vi "ustalRuchPionowy.vi"(6 "Kąt uśredniony":i32, 9 "Wybór komory":T3, 10 "Lista punktów w pionie":i32[](array[numeric]), 11 "Faza ruchu wstepna":T2) -> (2 "Stan pionowy":T1, 3 "Faza ruchu poziomego":T2)   [LabVIEW 2014]
uses:
  parametryKomorVIs/WyborKomory.ctl
  Faza_ruchu.ctl
  RuchPionowy.ctl
  AkcjaGFV.ctl
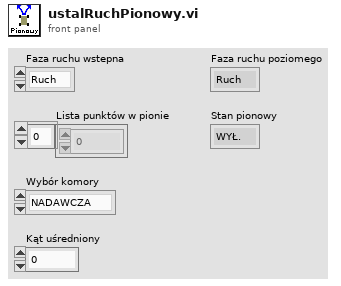
[diagram p1: front panel]
types:
  T1 = typedef "RuchPionowy.ctl" = enum16{"WYŁ.", "GÓRA", "Dӣ", "PRACA RĘCZNA"}
  T2 = typedef "Faza_ruchu.ctl" = enum16{"Ruch", "Poczekaj", "Pomiar"}
  T3 = typedef "WyborKomory.ctl" = enum16{"NADAWCZA", "ODBIORCZA"}
  T4 = typedef "WejsciaParametry.ctl" = cluster{"LEWO":bool, "PRAWO":bool, "GORA":bool, "DOL":bool, "Praca reczna":bool, "Stop":bool, "Start":bool, "Komora":bool, "Wyjscie":bool, "Rodzaj pomiarow":T5, "Czas pomiaru [s]":dbl, "Czas inicjalizacji ramion [s]":dbl, "Liczba punktów":i32, "Liczba płaszczyzn":i32}
  T5 = typedef "RodzajPomiarow.ctl" = enum16{"Izolacyjność Akustyczna ISO 10140", "Losowanie punktów", "Sekwencja testowa"}
  T6 = typedef "AkcjaGFV.ctl" = enum16{"Czytaj", "Zapisz", "Reset"}
  T7 = typedef "Gotowosc.ctl" = cluster{"Poziomy":bool, "Pionowy":bool}
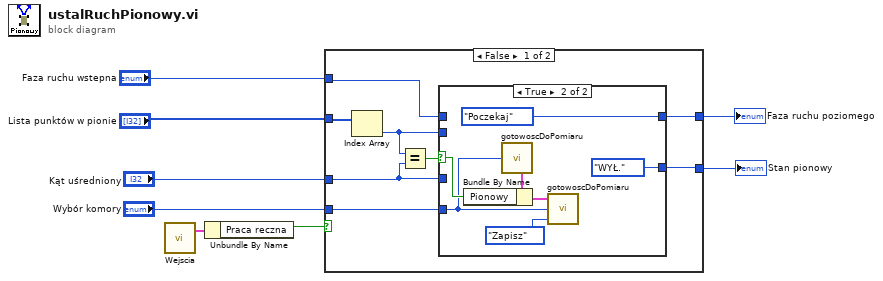
[diagram p0: block diagram]
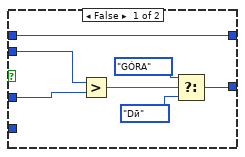
[diagram p2: hidden frame]
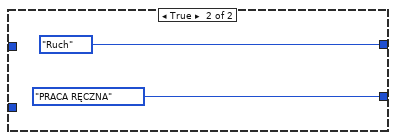
[diagram p3: hidden frame]
diagram:
  n1 = call "Wejscia.vi"() -> ("Wyjście"=w1:T4)  [unwired: 5 in]
  n2 = Unbundle By Name(w1) -> ("Praca reczna"=w2:bool)
  n3 = case shown="False" w2 {
    tunnel: "Kąt uśredniony" -> [w12 _]
    tunnel: [w14 RuchPionowy."PRACA RĘCZNA" ("Stan pionowy")] -> w3
    tunnel: "Faza ruchu wstepna" -> [w15 _]
    tunnel: [w16 Faza_ruchu."Ruch" ("Faza ruchu")] -> w5
    tunnel: "Lista punktów w pionie" -> [w11 _]
    tunnel: "Wybór komory" -> [w9 _]
    frame False {
      n4 = Index Array(array=w11) -> (element=w10:i32)  [unwired: 1 in]
      n5 = Equal?(x=w10, y=w12) -> (x = y?=w13:bool)
      n6 = case shown="True" w13 {
        selector: w13 -> [_ w26]
        tunnel: [w23 Faza_ruchu."Poczekaj" ("t")] -> w16
        tunnel: w15 -> [w23 _]
        tunnel: [w18 RuchPionowy."WYŁ." ("Stan pionowy")] -> w14
        tunnel: w12 -> [w22 _]
        tunnel: w10 -> [w17 _]
        tunnel: w9 -> [_ w24]
        frame False {
          n7 = Greater?(x=w17, y=w22) -> (0:w21:bool)
          n8 = Select(t=RuchPionowy."GÓRA" ("Stan pionowy"), s=w21, f=RuchPionowy."Dӣ") -> (s? t:f=w18:T1)
        }
        frame True {
          n9 = call "gotowoscDoPomiaru.vi"("Wybór komory"=w24) -> ("Gotowość wyjście"=w27:T7)  [unwired: 4 in]
          n10 = Bundle By Name(cluster=w27, "Pionowy"=w26) -> (w28:T7)
          n11 = call "gotowoscDoPomiaru.vi"("Akcja"=AkcjaGFV."Zapisz", "Wybór komory"=w24, "Gotowość"=w28) -> ()  [unwired: 2 in, 1 out]
        }
      }
    }
    frame True {
    }
  }
  "Faza ruchu poziomego" <- w5
  "Stan pionowy" <- w3
